vi "__uintCheckUintPair.vi"(8 "Error in (no error)":errorcluster, 10 "Uint2 in":refnum<class "UintClass.lvclass">, 11 "Uint1 in":refnum<class "UintClass.lvclass">) -> (0 "Error out":errorcluster, 1 "Timeout (-1)":T1=-1, 2 "Uint2 out":u8[](array[numeric]), 3 "Uint1 out":u8[](array[numeric]), 4 "Base out":T2=10 caption="Base (decimal)" items=["Binary"=2, "Octal"=8, "Decimal"=10, "Hexadecimal"=16, "Hexatrigesimal"=36, "ASCII"=64])   [LabVIEW 2011, in "UintClass.lvclass"]
uses:
  UintClass.lvclass
  enumBase.ctl
  timeout.ctl
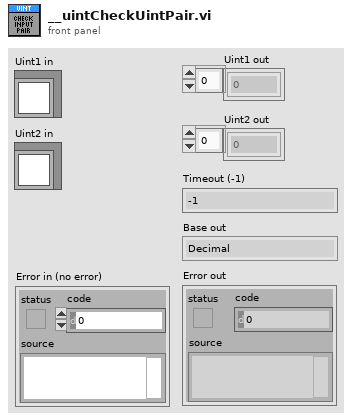
[diagram p1: front panel]
types:
  T1 = typedef "UintClass.lvclass/timeout.ctl" = i32
  T2 = typedef "UintClass.lvclass/enumBase.ctl" = u16
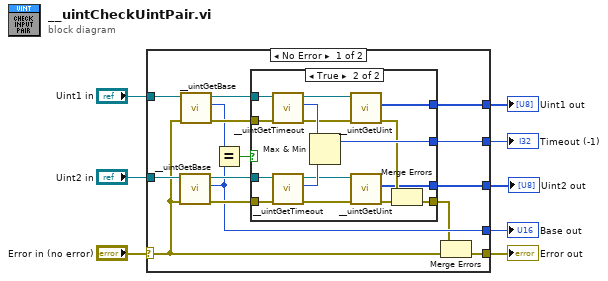
[diagram p0: block diagram]
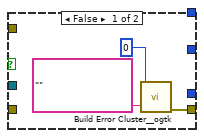
[diagram p2: hidden frame]
diagram:
  n1 = case shown="No Error" "Error in (no error)" {
    selector: "Error in (no error)" -> [w12 w43]
    tunnel: "Uint1 in" -> [w23 _]
    tunnel: "Uint2 in" -> [w22 _]
    tunnel: [w11 w43] -> w5
    tunnel: [w15 _] -> w2
    tunnel: [w14 _] -> w1
    tunnel: [w10 _] -> w4
    tunnel: [w9 _] -> w3
    frame No Error {
      n2 = call "__uintGetBase.vi"("Error in (no error)"=w12, "UintClass in"=w22) -> ("Error out"=w16:errorcluster, "Base (decimal)"=w15:T2, "UintClass out"=w17:refnum<class "UintClass.lvclass">)  [unwired: 7 in]
      n3 = call "__uintGetBase.vi"("Error in (no error)"=w12, "UintClass in"=w23) -> ("Error out"=w20:errorcluster, "Base (decimal)"=w18:T2, "UintClass out"=w21:refnum<class "UintClass.lvclass">)  [unwired: 7 in]
      n4 = Equal?(x=w18, y=w15) -> (x = y?=w19:bool)
      n5 = case shown="True" w19 {
        tunnel: w21 -> [_ w42]
        tunnel: w20 -> [_ w41]
        tunnel: w17 -> [_ w40]
        tunnel: w16 -> [_ w39]
        tunnel: [_ w36] -> w14
        tunnel: [w26 w29] -> w13
        tunnel: [_ w28] -> w10
        tunnel: [_ w27] -> w9
        frame False {
          n6 = call <userlib>:"Build Error Cluster__ogtk.vi"("String to Prepend to source (\"\")"="" ("String to Prepend to source (\"\")"), "code"=0) -> ("error out"=w26:errorcluster)
        }
        frame True {
          n7 = call "__uintGetTimeout.vi"("Error in (no error)"=w41, "UintClass in"=w42) -> ("Error out"=w33:errorcluster, "Timeout (-1)"=w38:T1, "UintClass out"=w32:refnum<class "UintClass.lvclass">)  [unwired: 7 in]
          n8 = call "__uintGetTimeout.vi"("Error in (no error)"=w39, "UintClass in"=w40) -> ("Error out"=w34:errorcluster, "Timeout (-1)"=w37:T1, "UintClass out"=w35:refnum<class "UintClass.lvclass">)  [unwired: 7 in]
          n9 = Max & Min(x=w38, y=w37) -> (max(x,y)=w36:T1)  [unwired: 1 out]
          n10 = call "__uintGetUint.vi"("Error in (no error)"=w33, "UintClass in"=w32) -> ("Error out"=w31:errorcluster, "Uint (0)"=w28:u8[])  [unwired: 7 in, 1 out]
          n11 = call "__uintGetUint.vi"("Error in (no error)"=w34, "UintClass in"=w35) -> ("Error out"=w30:errorcluster, "Uint (0)"=w27:u8[])  [unwired: 7 in, 1 out]
          n12 = Merge Errors(w31, w30) -> (w29:errorcluster)
        }
      }
      n13 = Merge Errors(w13, w12) -> (w11:errorcluster)
    }
    frame Error {
    }
  }
  "Error out" <- w5
  "Uint1 out" <- w4
  "Uint2 out" <- w3
  "Base out" <- w2
  "Timeout (-1)" <- w1
